vi "DIOSerialPortTx.vi"(11 "DIOSerialPortSettings":T1={"TxPort"="ModbusPort1Tx", "TxDataFIFO"="ModbusPort1TxFIFO", "RxPort"="ModbusPort1Rx", "RxDataFIFO"="ModbusPort1RxFIFO"}) -> ()   [LabVIEW 2016]
uses:
  DIOSerialPortSettings.ctl
  DIOSerialPortTxData.ctl
  DIOSerialPortTxStates.ctl
  <vilib>/Platform/TimedLoop/XDataNode/timing_clust.ctl
  <vilib>/Platform/TimedLoop/XDataNode/nitl_modes.ctl
  <vilib>/Platform/TimedLoop/XDataNode/wakeup.ctl
  <vilib>/rvi/Emulation/niFpgaSctlEmulationGetInTimedLoop.vi
  <vilib>/rvi/Emulation/niFpgaEmulationReportErrorSimple.vi
  <vilib>/rvi/Emulation/niFpgaGetClockAttributes.vi
  <vilib>/rvi/Emulation/niFpgaCriticalErrorInLSC.vi
  <vilib>/rvi/DataTransferAndStorage/Container/Common/niFpgaContainerExecOnDevCompGetState.vi
  <vilib>/rvi/Emulation/niFpgaEmulationIsFPGAContextNoSignature.vi
  <vilib>/rvi/errors/niFpgaSetErrorForExecOnDevCompSimple.vi
  <vilib>/rvi/eio/common/nirviEmuReportErrorAndStop.vi
  <vilib>/rvi/DataTransferAndStorage/Container/Common/niFpgaContainerGetUniqueNameForEmu.vi
  <vilib>/rvi/FIFO/Fifo_Resource/nirvififoEmulationSetSize.vi
  <vilib>/rvi/FIFO/Fifo_Resource/nirviFifoEmulationQueueMgr.vi
  <instcachedir>/0/nirviFifoEmulationQueueMgr_E5CAEC123FF24DC58D834DCA3CDAA9B5.lvgen/nirviFifoEmulationQueueMgr_E5CAEC123FF24DC58D834DCA3CDAA9B5_009.vi
  <vilib>/rvi/FIFO/Fifo_Resource/nirvififoEmulationDetermineInputValidOut.vi
  <vilib>/rvi/FIFO/Fifo_Resource/nirvififoEmulationCreateLock.vi
  <vilib>/rvi/Emulation/niFpgaProcessEmulError.vi
  <vilib>/rvi/FIFO/Fifo_Resource/nirvififoEmulationObtainLock.vi
  <vilib>/rvi/FIFO/Fifo_Resource/nirvififoEmulationReleaseLock.vi
  <vilib>/rvi/occurrence/nirviWaitOnOccurrenceBase.vi
  <vilib>/rvi/errors/nirviReportUnexpectedCaseInternalError.vi
  <vilib>/rvi/errors/nirviReportUnexpectedCaseInternalError (U32).vi
  <vilib>/Utility/error.llb/Clear Errors.vi
  <vilib>/rvi/interface/RandomDataEmulation/niFpgaRandomDataHandleErrors.vi
  <vilib>/rvi/eio/common/nirviEmuTemplateMethod_errors.vi
  <vilib>/Platform/TimedLoop/XDataNode/XDataNode.xnode
  <vilib>/rvi/DataTransferAndStorage/Container/XNode/niFpgaContainer.xnode
  <vilib>/rvi/FIFO/Fifo_Resource/niFpgaFifoEmulationRefIn.vi
  <vilib>/eio/EIONode/EIONode.xnode
  <vilib>/Platform/TimedLoop/XDataNode/XDNodeRunTimeDep.lvlib
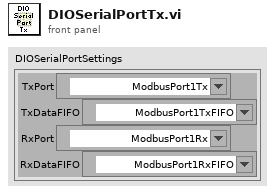
[diagram p1: front panel]
types:
  T1 = typedef "DIOSerialPortSettings.ctl" = cluster{"TxPort":refnum<k21>, "TxDataFIFO":refnum<k21>, "RxPort":refnum<k21>, "RxDataFIFO":refnum<k21>}
  T2 = typedef "DIOSerialPortTxData.ctl" = cluster{"State":T3, "DelayTicks":u8, "StateAfterDelay":T3, "Data":u8, "Bit":u8}
  T3 = typedef "DIOSerialPortTxStates.ctl" = enum16{"ReadByte", "WriteStartBit", "WriteDataBits", "WriteStopBit", "Delay"}
  T4 = typedef "XDNodeRunTimeDep.lvlib/timing_clust.ctl" = cluster{"Expected End [f-1]":u64, "Actual End [f-1]":u64, "Finished Late? [f-1]":bool, "Expected End [i-1]":u64, "Actual End [i-1]":u64, "Finished Late? [i-1]":bool, "Expected Start [i]":u64, "Actual Start [i]":u64, "Expected Start [f]":u64, "Actual Start [f]":u64, "Source Name":string, "Structure Name":string, "Period":i64, "Deadline":i64, "Offset":i64, "Start":i64, "Priority":i32, "Timeout":i32, "Mode":T5, "Wakeup Reason":T6, "Error":errorcluster, "Source Type":string, "Secondary Source Type":string, "Global End Time":u64, "Global Start Time":u64, "Frame Duration":u64, "Iteration Duration":u64, "Assigned CPU":i32, "I/O Scan Engine Mode":u32}
  T5 = typedef "XDNodeRunTimeDep.lvlib/nitl_modes.ctl" = enum32{"No Change", "Process missed periods, maintain original phase", "Discard missed periods, maintain original phase", "Process missed periods, ignore original phase", "Discard missed periods, ignore original phase"}
  T6 = typedef "XDNodeRunTimeDep.lvlib/wakeup.ctl" = enum32{"Normal", "Aborted", "Asynchronous wakeup", "Timing source error", "Timed loop error", "Timeout"}
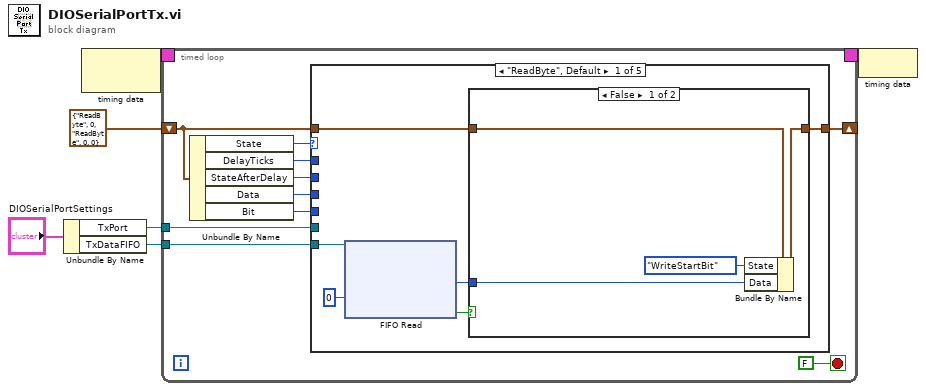
[diagram p0: block diagram]
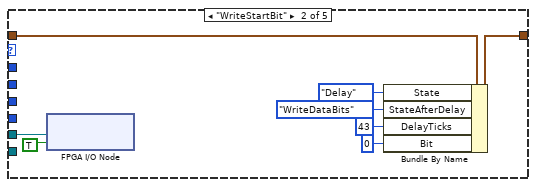
[diagram p3: hidden frame]
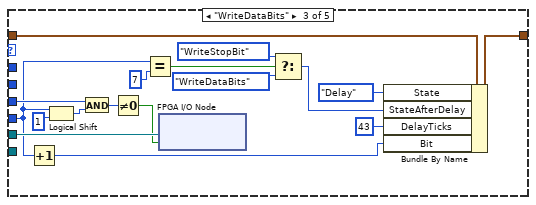
[diagram p4: hidden frame]
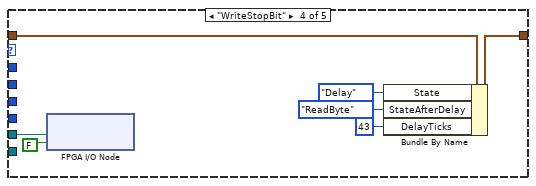
[diagram p5: hidden frame]
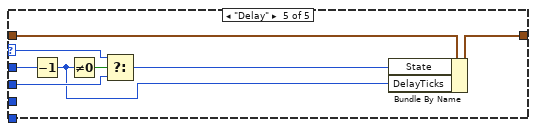
[diagram p6: hidden frame]
diagram:
  n1 = Unbundle By Name("DIOSerialPortSettings") -> ("TxPort"=w2:refnum<k21>, "TxDataFIFO"=w1:refnum<k21>)
  n2 = node-c288() -> (w6:T4)  [unwired: 1 in]
  n3 = timed-loop {
    timing: w6 -> [_]
    timing-out: [_] -> w5
    shift-right: [w15] -> _
    shift-left: T2 {"State"=enum."ReadByte", "DelayTicks"=0, "StateAfterDelay"=enum."ReadByte", "Data"=0, "Bit"=0} ("DIOSerialPortTxData") -> [w16]
    tunnel: w2 -> [w8]
    tunnel: w1 -> [w13]
    stop <- FALSE stop-if-true
    n4 = Unbundle By Name(w16) -> ("State"=w14:T3, "DelayTicks"=w12:u8, "StateAfterDelay"=w11:T3, "Data"=w10:u8, "Bit"=w9:u8)
    n5 = case shown="\"ReadByte\", Default" w14 {
      selector: w14 -> [_ _ _ _ w63]
      tunnel: w16 -> [w19 w35 w52 w59 w67]
      tunnel: [w18 w34 w51 w58 w66] -> w15
      tunnel: w13 -> [w22 _ _ _ _]
      tunnel: w12 -> [_ _ _ _ w65]
      tunnel: w11 -> [_ _ _ _ w62]
      tunnel: w10 -> [_ _ w45 _ _]
      tunnel: w9 -> [_ _ w40 _ _]
      tunnel: w8 -> [_ w29 w48 w54 _]
      frame "ReadByte", Default {
        n6 = xnode "FIFO Read"("Timeout"=0, "FIFO In"=w22) -> ("Element"=w17:u8, "Timed Out?"=w20:bool)  [unwired: 1 out]
        n7 = case shown="False" w20 {
          tunnel: w19 -> [w26 w27]
          tunnel: [w25 w27] -> w18
          tunnel: w17 -> [w23 _]
          frame False {
            n8 = Bundle By Name(cluster=w26, "State"=DIOSerialPortTxStates."WriteStartBit", "Data"=w23) -> (w25:T2)
          }
          frame True {
          }
        }
      }
      frame "WriteStartBit" {
        n9 = xnode "FPGA I/O Node"("I/O Item"=TRUE, "FPGA I/O In"=w29) -> ()  [unwired: 1 out]
        n10 = Bundle By Name(cluster=w35, "State"=DIOSerialPortTxStates."Delay", "StateAfterDelay"=DIOSerialPortTxStates."WriteDataBits", "DelayTicks"=u8 43, "Bit"=u8 0) -> (w34:T2)
      }
      frame "WriteDataBits" {
        n11 = Increment(x=w40) -> (x+1=w47:u8)
        n12 = Logical Shift(y=w40, x=i16 1) -> (x << y=w43:i16)
        n13 = And(x=w45, y=w43) -> (x .and. y?=w44:i16)
        n14 = Not Equal To 0?(x=w44) -> (x != 0?=w42:bool)
        n15 = Equal?(x=w40, y=i16 7) -> (x = y?=w39:bool)
        n16 = xnode "FPGA I/O Node"("I/O Item"=w42, "FPGA I/O In"=w48) -> ()  [unwired: 1 out]
        n17 = Select(t=DIOSerialPortTxStates."WriteStopBit" ("StateAfterDelay"), s=w39, f=DIOSerialPortTxStates."WriteDataBits" ("StateAfterDelay")) -> (s? t:f=w36:T3)
        n18 = Bundle By Name(cluster=w52, "State"=DIOSerialPortTxStates."Delay", "StateAfterDelay"=w36, "DelayTicks"=u8 43, "Bit"=w47) -> (w51:T2)
      }
      frame "WriteStopBit" {
        n19 = xnode "FPGA I/O Node"("I/O Item"=FALSE, "FPGA I/O In"=w54) -> ()  [unwired: 1 out]
        n20 = Bundle By Name(cluster=w59, "State"=DIOSerialPortTxStates."Delay", "StateAfterDelay"=DIOSerialPortTxStates."ReadByte", "DelayTicks"=u8 43) -> (w58:T2)
      }
      frame "Delay" {
        n21 = Decrement(x=w65) -> (x-1=w60:u8)
        n22 = Not Equal To 0?(x=w60) -> (x != 0?=w64:bool)
        n23 = Select(t=w63, s=w64, f=w62) -> (s? t:f=w61:T3)
        n24 = Bundle By Name(cluster=w67, "State"=w61, "DelayTicks"=w60) -> (w66:T2)
      }
    }
  }
  n25 = node-c288(w5) -> ()
